vi "PM5000_Waveform_Log.vi"(8 "error in":errorcluster, 11 "Network Path":string="172.22.26.202") -> (0 "error out":errorcluster, 3 "Network Path out":string="192.168.169.1")   [LabVIEW 2018]
doc: "Lee la tabla de memoria RealTime_VIF_Power del equipo PowerMonitor 5000, ademas filtra y ordena las variables de interez de la tabla de memoria.\n\nLee las siguientes variables de la tabla RealTime_VIF_Power:\n\n*V1_V2_Volts\n*V2_V3_Volts\n*V3_V1_Volts\n*I1_Amps\n*I2_Amps\n*I3_Amps\n*Frequency_Hz\n*Total_kW\n*Total_kVAR\n*Total_kVA\n*Total_True_PF\n*Total_Disp_PF"
uses:
  <vilib>/ethernetip/ethernetip.llb/EthernetIP SLC500 Read Float.vi
  <vilib>/ethernetip/ethernetip.lvlib
panel:
  out "Data":sgl[](array[numeric])
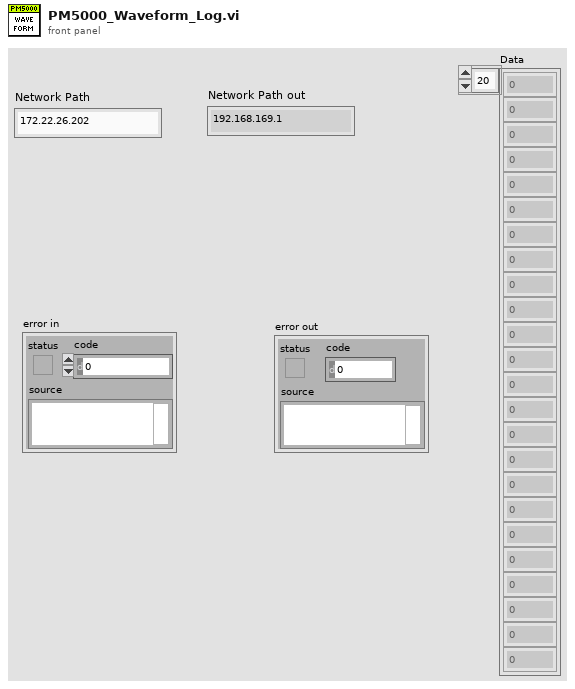
[diagram p1: front panel]
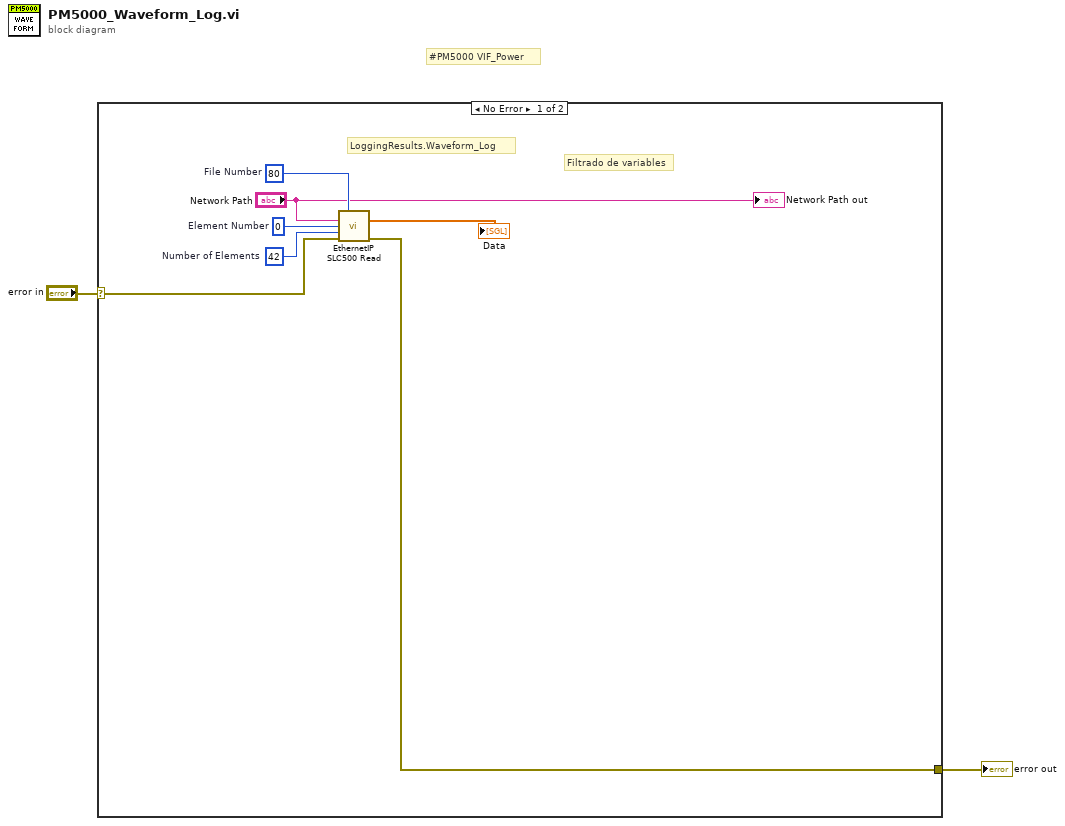
[diagram p0: block diagram]
diagram:
  # "#PM5000 VIF_Power"
  n1 = case shown="No Error" "error in" {
    selector: "error in" -> [w4 w10]
    tunnel: [w6 w10] -> w2
    frame No Error {
      w7 = u32 42  # Number of Elements
      w9 = u16 80  # File Number
      w8 = u16 0  # Element Number
      # "Filtrado de variables"
      # "LoggingResults.Waveform_Log"
      n2 = call-poly <vilib>:"EthernetIP SLC500 Read.vi"("File Number"=w9, "Network Path"="Network Path", "Element Number"=w8, "Number of Elements"=w7, "error in"=w4) -> ("Data"=→"Data":sgl[], "error out"=w6:errorcluster)  [unwired: 8 in, 1 out]
      "Network Path out" <- "Network Path"
    }
    frame Error {
    }
  }
  "error out" <- w2
